vi "HEAD.vi"(6 "timeout":i32=10000, 8 "error in":errorcluster, 10 "url":string, 11 "http-client in":refnum<class "http-client.lvclass">) -> (0 "error out":errorcluster, 2 "headers":string, 3 "http-client out":refnum<class "http-client.lvclass">, 4 "status code":u16)   [LabVIEW 2025, in "http-client.lvclass"]
uses:
  http-client.lvclass
  REST Client/REST Client.lvclass
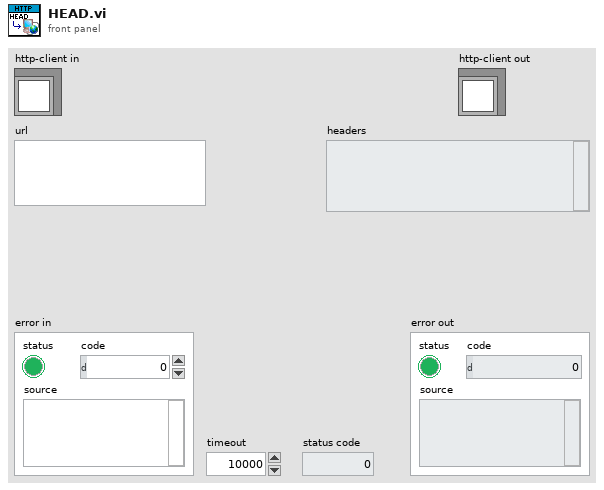
[diagram p1: front panel]
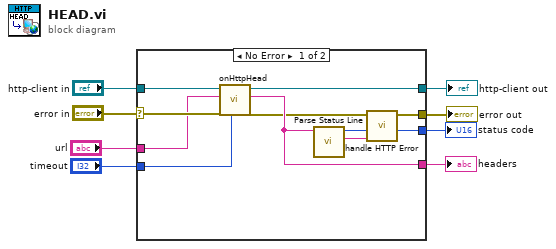
[diagram p0: block diagram]
diagram:
  n1 = case shown="No Error" "error in" {
    selector: "error in" -> [w17 w21]
    tunnel: [w12 w21] -> w7
    tunnel: [w19 w20] -> w5
    tunnel: "http-client in" -> [w18 w20]
    tunnel: [w14 _] -> w4
    tunnel: "url" -> [w16 _]
    tunnel: "timeout" -> [w15 _]
    tunnel: [w9 _] -> w1
    frame No Error {
      n2 = call-dynamic "onHttpHead.vi"("timeout"=w15, "error in"=w17, "url"=w16, "http-method in"=w18) -> ("error out"=w13:errorcluster, "headers"=w14:string, "http-method out"=w19:refnum<class "http-client.lvclass">)  [unwired: 5 in]
      n3 = call "Parse Status Line.vi"("Headers w/ status line"=w14) -> ("Status String"=w10:string, "status code"=w11:u16)  [unwired: 6 in, 3 out]
      n4 = call "handle HTTP Error.vi"("Status String"=w10, "status code"=w11, "error in (no error)"=w13) -> ("status code dup"=w9:u16, "error out"=w12:errorcluster)  [unwired: 7 in]
    }
    frame Error {
    }
  }
  "error out" <- w7
  "http-client out" <- w5
  "headers" <- w4
  "status code" <- w1
